vi "Execute.vi"(0 "reference in":refnum<class "MacroCommand.lvclass">, 5 "error in (no error)":errorcluster) -> (14 "reference out":refnum<class "MacroCommand.lvclass">, 19 "error out":errorcluster)   [LabVIEW 2013, in "MacroCommand.lvclass"]
uses:
  MacroCommand.lvclass
  Command_class/Command.lvclass
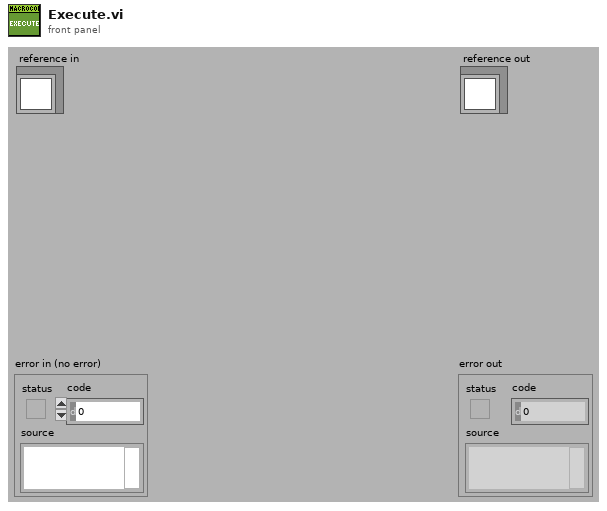
[diagram p1: front panel]
types:
  T1 = typedef "MacroCommand.lvclass/ObjectAttributes.ctl" = cluster{"Command Array":refnum<class "Command.lvclass">[]}
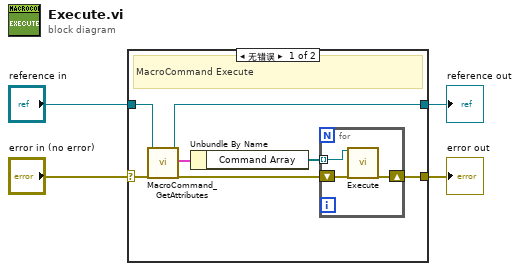
[diagram p0: block diagram]
diagram:
  n1 = case shown="无错误" "error in (no error)" {
    selector: "error in (no error)" -> [w11 w16]
    tunnel: [w5 w16] -> w3
    tunnel: [w10 w15] -> w1
    tunnel: "reference in" -> [w8 w15]
    frame No Error {
      # "MacroCommand Execute"
      n2 = call "MacroCommand_GetAttributes.vi"("reference in"=w8, "error in (no error)"=w11) -> ("reference out"=w10:refnum<class "MacroCommand.lvclass">, "attributes"=w9:T1, "error out"=w6:errorcluster)  [unwired: 14 in, 1 out]
      n3 = Unbundle By Name(w9) -> ("Command Array"=w7:refnum<class "Command.lvclass">[])
      n4 = for {
        tunnel: w7 -> [w14] mode=indexing
        shift-right: [w12] -> w5
        shift-left: w6 -> [w13]
        n5 = call-dynamic "Execute.vi"("reference in"=w14, "error in (no error)"=w13) -> ("error out"=w12:errorcluster)  [unwired: 16 in, 1 out]
      }
    }
    frame Error {
    }
  }
  "error out" <- w3
  "reference out" <- w1
